vi "Interface.RT FIFO.Create.vi"   [LabVIEW 2017, in "DSF Core.lvlib" / "Interface.lvclass"]
uses:
  Interface.lvclass
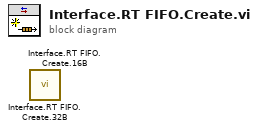
[diagram p0: block diagram]
diagram:
  n1 = call "Interface.RT FIFO.Create.32B.vi"() -> ()  [unwired: 10 in, 2 out]
  n2 = call "Interface.RT FIFO.Create.16B.vi"() -> ()  [unwired: 10 in, 2 out]
